vi "File.Find Path from Abs-Relative Path.vi"(7 "Search Folders":path[](array[path]), 10 "error in (no error)":errorcluster, 11 "Rel Path":string) -> (2 "error out":errorcluster, 3 "Path":path)   [LabVIEW 2024, in "EQMF.lvlib" / "File Utils.lvlib"]
uses:
  File Utils.lvlib
panel:
  out "Rel":bool
  out "Abs":bool
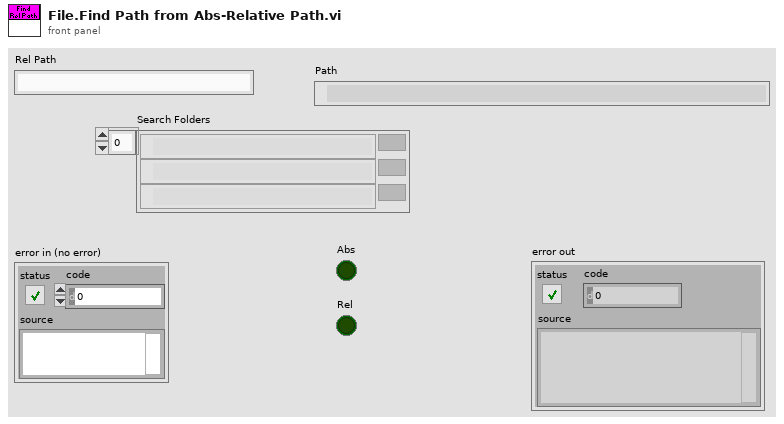
[diagram p1: front panel]
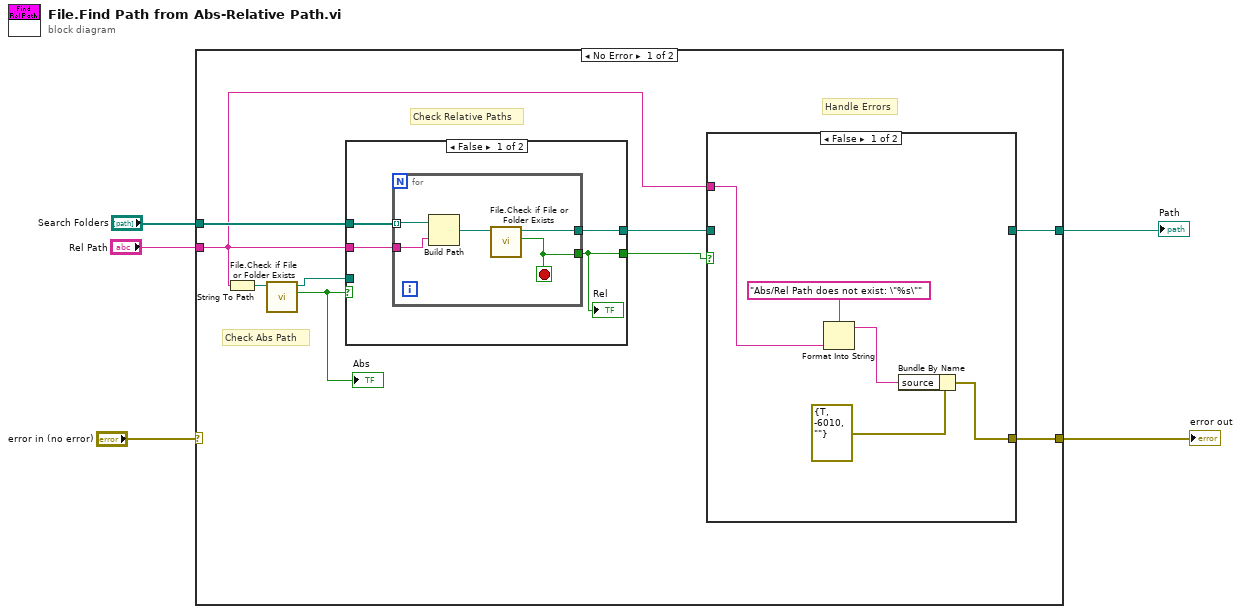
[diagram p0: block diagram]
diagram:
  n1 = case shown="No Error" "error in (no error)" {
    selector: "error in (no error)" -> [_ w32]
    tunnel: [w9 w32] -> w4
    tunnel: "Rel Path" -> [w7 _]
    tunnel: "Search Folders" -> [w13 _]
    tunnel: [w10 _] -> w1
    frame No Error {
      # "Handle Errors"
      # "Check Abs Path"
      # "Check Relative Paths"
      n2 = String To Path(string=w7) -> (path=w14:path)
      n3 = call "File.Check if File or Folder Exists.vi"("Path"=w14) -> ("Exists"=w6:bool, "Dup Path"=w12:path)  [unwired: 6 in, 3 out]
      "Abs" <- w6
      n4 = case shown="False" w6 {
        selector: w6 -> [_ w31]
        tunnel: w13 -> [w24 _]
        tunnel: w7 -> [w23 _]
        tunnel: [w22 w30] -> w11
        tunnel: w12 -> [_ w30]
        tunnel: [w21 w31] -> w8
        frame False {
          n5 = for {
            tunnel: w24 -> [w29] mode=indexing
            tunnel: w23 -> [w28]
            tunnel: [w26] -> w22
            tunnel: [w25] -> w21
            stop <- w25 stop-if-true
            n6 = Build Path(base path=w29, name or relative path=w28) -> (appended path=w27:path)
            n7 = call "File.Check if File or Folder Exists.vi"("Path"=w27) -> ("Exists"=w25:bool, "Dup Path"=w26:path)  [unwired: 6 in, 3 out]
          }
          "Rel" <- w21
        }
        frame True {
        }
      }
      n8 = case shown="False" w8 {
        tunnel: w11 -> [_ w20]
        tunnel: [_ w20] -> w10
        tunnel: [w16 _] -> w9
        tunnel: w7 -> [w15 _]
        frame False {
          n9 = Format Into String(format string="Abs/Rel Path does not exist: \"%s\"", w15) -> (resulting string=w17:string)  [unwired: 2 in, 1 out]
          n10 = Bundle By Name(cluster=errorcluster {"status"=TRUE, "code"=-6010, "source"=""} ("error constant"), "source"=w17) -> (w16:errorcluster)
        }
        frame True {
        }
      }
    }
    frame Error {
    }
  }
  "Path" <- w1
  "error out" <- w4
